vi "GP275.vi"() -> ()   [LabVIEW 2011]
panel:
  out "Numeric 2":u16 format="%x"
  out "Numeric":u16
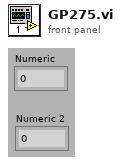
[diagram p1: front panel]
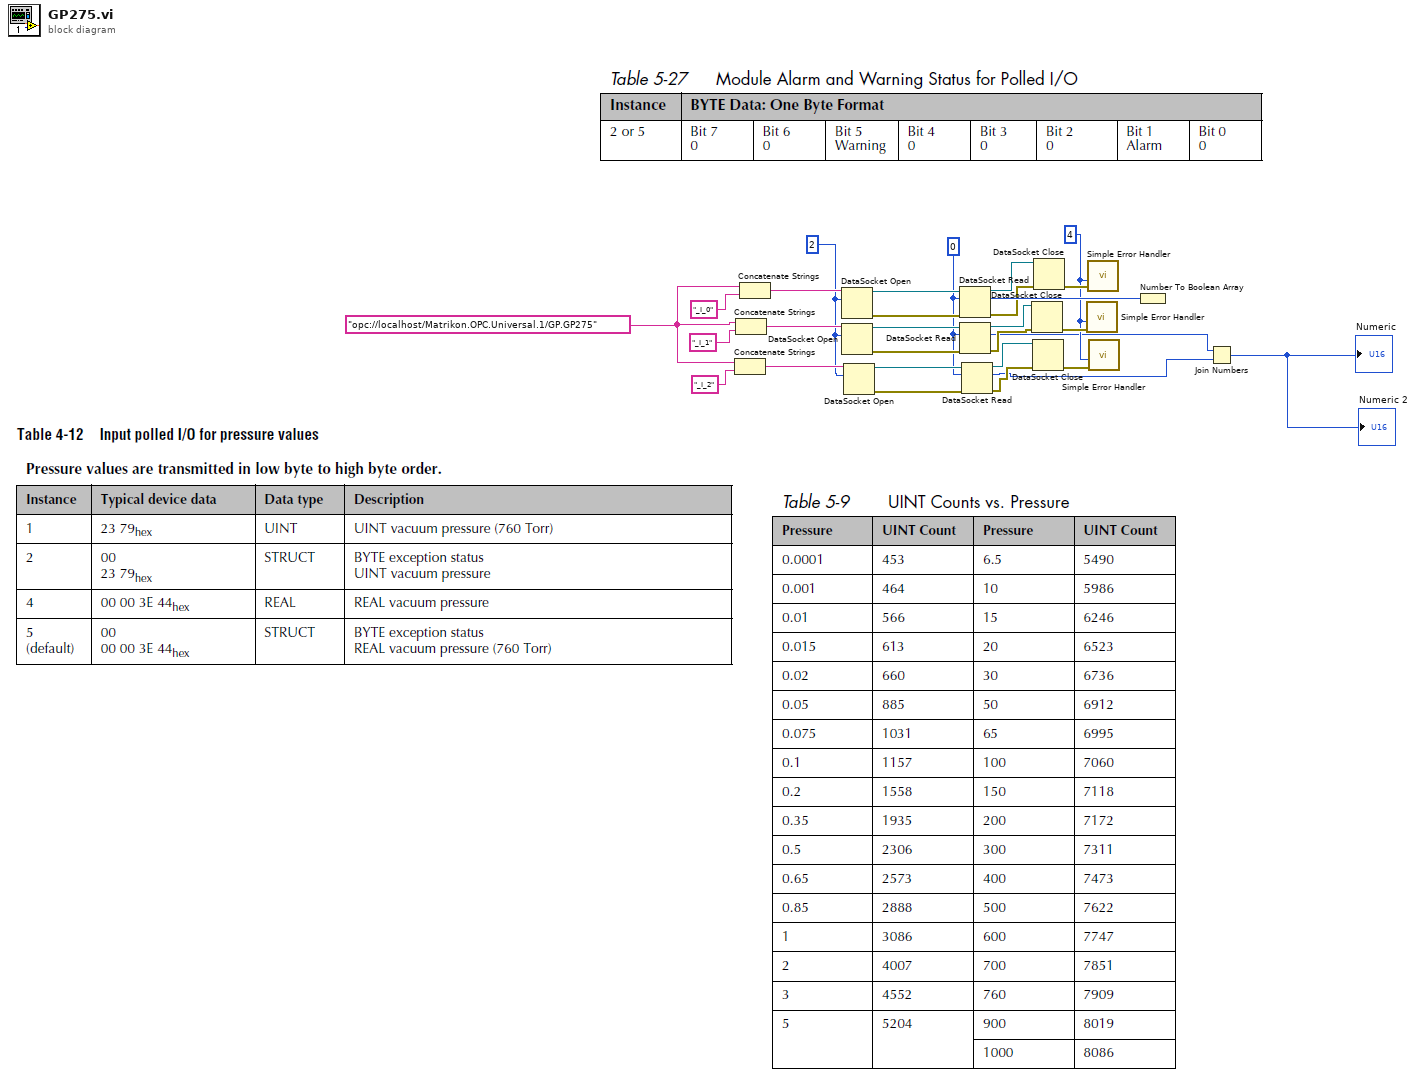
[diagram p0: block diagram]
diagram:
  w5 = 4
  w13 = i8 0
  w14 = 2
  w4 = "opc://localhost/Matrikon.OPC.Universal.1/GP.GP275"
  n1 = Concatenate Strings(w4, "_I_2") -> (w21:string)
  n2 = Concatenate Strings(w4, "_I_1") -> (w22:string)
  n3 = Concatenate Strings(w4, "_I_0") -> (w23:string)
  n4 = DataSocket Open(10:w14, 11:w23) -> (0:w18:errorcluster, 3:w26:refnum<k13>)  [unwired: 2 in]
  n5 = DataSocket Open(10:w14, 11:w22) -> (0:w19:errorcluster, 3:w25:refnum<k13>)  [unwired: 2 in]
  n6 = DataSocket Open(10:w14, 11:w21) -> (0:w20:errorcluster, 3:w24:refnum<k13>)  [unwired: 2 in]
  n7 = DataSocket Read(8:w18, 10:w13, 11:w26) -> (0:w9:errorcluster, 2:w12:i8, 3:w17:refnum<k13>)  [unwired: 2 in, 4 out]
  n8 = DataSocket Read(8:w19, 10:w13, 11:w25) -> (0:w10:errorcluster, 2:w1:i8, 3:w16:refnum<k13>)  [unwired: 2 in, 4 out]
  n9 = DataSocket Read(8:w20, 10:w13, 11:w24) -> (0:w11:errorcluster, 2:w2:i8, 3:w15:refnum<k13>)  [unwired: 2 in, 4 out]
  n10 = DataSocket Close(8:w10, 11:w16) -> (0:w7:errorcluster)  [unwired: 1 in, 1 out]
  n11 = DataSocket Close(8:w11, 11:w15) -> (0:w6:errorcluster)  [unwired: 1 in, 1 out]
  n12 = DataSocket Close(8:w9, 11:w17) -> (0:w8:errorcluster)  [unwired: 1 in, 1 out]
  n13 = call <vilib>:"Simple Error Handler.vi"("type of dialog (OK msg:1)"=w5, "error in (no error)"=w7) -> ()  [unwired: 3 in, 5 out]
  n14 = call <vilib>:"Simple Error Handler.vi"("type of dialog (OK msg:1)"=w5, "error in (no error)"=w8) -> ()  [unwired: 3 in, 5 out]
  n15 = call <vilib>:"Simple Error Handler.vi"("type of dialog (OK msg:1)"=w5, "error in (no error)"=w6) -> ()  [unwired: 3 in, 5 out]
  n16 = Number To Boolean Array(number=w12) -> ()  [unwired: 1 out]
  n17 = Join Numbers(hi=w1, lo=w2) -> ((hi.lo)=→"Numeric" →"Numeric 2":u16)
